vi "1-2.vi"() -> ()   [LabVIEW 2019, in "1.lvlib"]
uses:
  <vilib>/Utility/file.llb/Read Delimited Spreadsheet (I64).vi
  1.lvlib
panel:
  out "index":i32
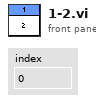
[diagram p1: front panel]
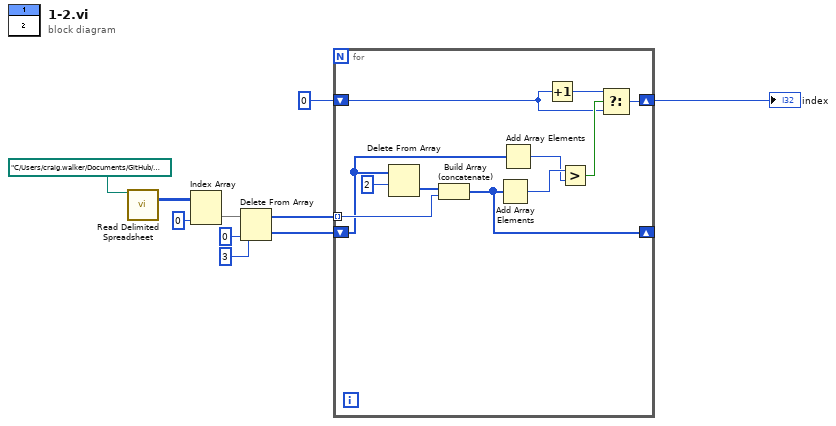
[diagram p0: block diagram]
diagram:
  n1 = call-poly <vilib>:"Read Delimited Spreadsheet.vi"("file path (dialog if empty)"=path "C:/Users/craig.walker/Documents/GitHub/lv2019-Advent-of-Code-2021/1/input.txt") -> ("all rows"=w9:i64[][])  [unwired: 9 in, 5 out]
  n2 = Index Array(array=w9, index (col)=0 ("disabled index (col)")) -> (element=w5:i64[])  [unwired: 1 in]
  n3 = Delete From Array(array=w5, length=3, index=0) -> (deleted portion=w1:i64[], array with subset deleted=w4:i64[])
  n4 = for {
    shift-right: [w20] -> w6
    shift-left: 0 ("index") -> [w18]
    tunnel: w4 -> [w17] mode=indexing
    shift-right: [w13] -> _
    shift-left: w1 -> [w12]
    n5 = Delete From Array(array=w12, length=2) -> (deleted portion=w11:i64[])  [unwired: 1 in, 1 out]
    n6 = Build Array (concatenate)(w11, w17) -> (w13:i64[])
    n7 = Add Array Elements(numeric array=w13) -> (sum=w16:i64)
    n8 = Add Array Elements(numeric array=w12) -> (sum=w15:i64)
    n9 = Increment(x=w18) -> (x+1=w19:i32)
    n10 = Greater?(x=w16, y=w15) -> (0:w21:bool)
    n11 = Select(t=w19, s=w21, f=w18) -> (s? t:f=w20:i32)
  }
  "index" <- w6
